vi "LVClasse_SurfaceFloat dtor.vi"(0 "SurfaceFloat in":refnum<class "SurfaceFloat.lvclass">, 11 "error in (no error)":errorcluster) -> (4 "SurfaceFloat out":refnum<class "SurfaceFloat.lvclass">, 15 "error out":errorcluster)   [LabVIEW 2020, in "SurfaceFloat.lvclass"]
doc: "Surface destructor.\n\n--------------------------------------------------------------------------------\n\n<B>surfaceIn </B> : Surface object.\n<B>surfaceOut </B> : Surface object.\n<B>ErrorIn </B> : Error\n<B>ErrorOut </B> : Error\n\n--------------------------------------------------------------------------------"
uses:
  SurfaceFloat.lvclass
  SurfaceFloat.lvclass/SurfaceFloat.ctl
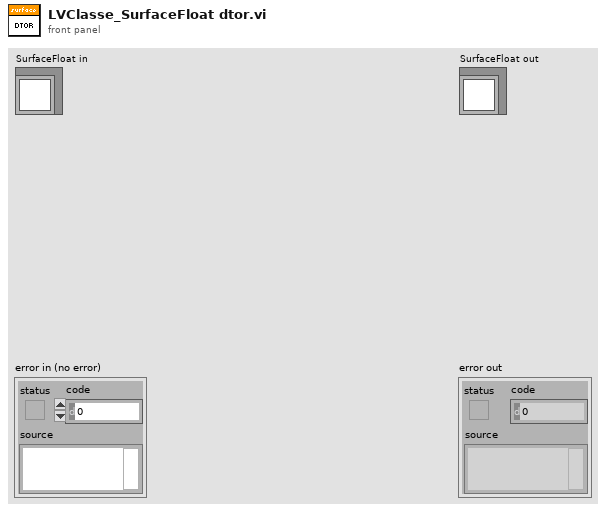
[diagram p1: front panel]
types:
  T1 = typedef "Handle creation.ctl" = enum16{"By ctor", "By write function"}
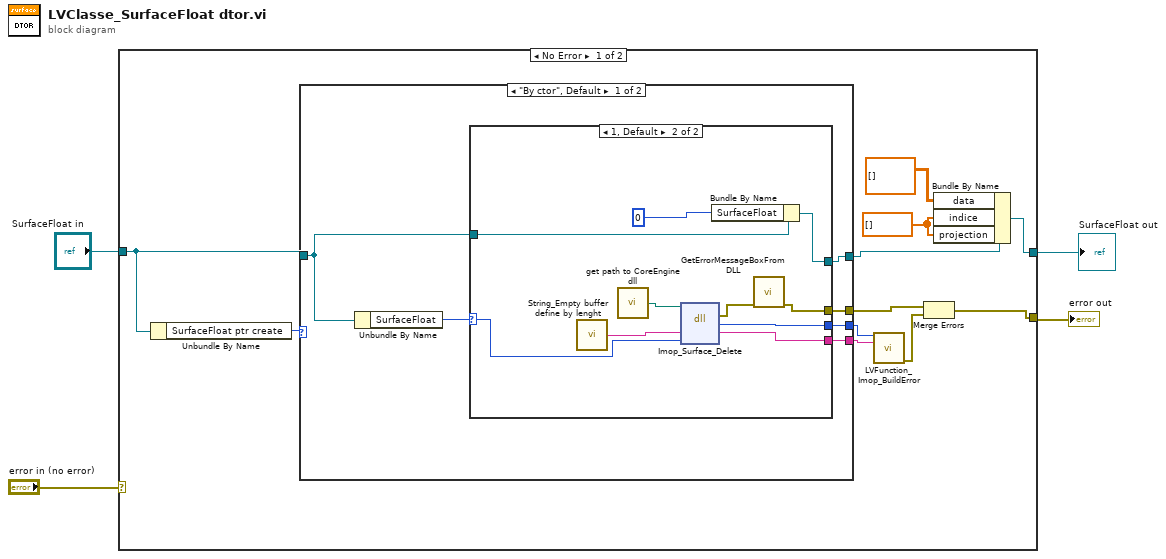
[diagram p0: block diagram]
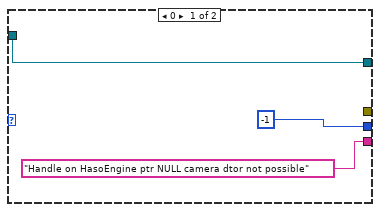
[diagram p2: hidden frame]
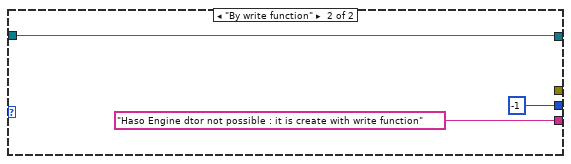
[diagram p3: hidden frame]
diagram:
  n1 = case shown="No Error" "error in (no error)" {
    selector: "error in (no error)" -> [_ w38]
    tunnel: "SurfaceFloat in" -> [w13 w39]
    tunnel: [w8 w39] -> w2
    tunnel: [w9 w38] -> w1
    frame No Error {
      w6 = sgl[] [] ("indice")
      n2 = Unbundle By Name(w13) -> ("SurfaceFloat ptr create"=w12:T1)
      n3 = case shown="\"By ctor\", Default" w12 {
        tunnel: [w21 "Haso Engine dtor not possible : it is create with write function" ("message")] -> w15
        tunnel: [w20 -1] -> w14
        tunnel: w13 -> [w18 w35]
        tunnel: [w19 w35] -> w7
        tunnel: [w16 _] -> w11
        frame "By ctor", Default {
          n4 = Unbundle By Name(w18) -> ("SurfaceFloat"=w17:i32)
          n5 = case shown="1, Default" w17 {
            selector: w17 -> [_ w31]
            tunnel: ["Handle on HasoEngine ptr NULL camera dtor not possible" ("message") w33] -> w21
            tunnel: [-1 w32] -> w20
            tunnel: w18 -> [w22 w27]
            tunnel: [w22 w26] -> w19
            tunnel: [_ w25] -> w16
            frame 0 {
            }
            frame 1, Default {
              n6 = call "String_Empty buffer define by lenght.vi"() -> ("Empty buffer"=w34:string)  [unwired: 1 in]
              n7 = call "get path to CoreEngine dll.vi"() -> ("path to c_interface_vc100.dll"=w30:path)  [unwired: 12 in, 3 out]
              n8 = dll-call lib="D:/soft/HASO_v3/SVN_trunk/ImOpCoreEngine4_LV2011/DLLs/c_interface_vc100.dll" fn="Imop_Surface_Delete"(path in=w30, "message"=w34, "surface"=w31) -> (error out=w29:errorcluster, "return type"=w32:i32, "message"=w33:string)  [unwired: 3 in, 1 out]
              n9 = Bundle By Name(cluster=w27, "SurfaceFloat"=u32 0 ("HasoEgine")) -> (w26:refnum<class "SurfaceFloat.lvclass">)
              n10 = call "GetErrorMessageBoxFromDLL.vi"("error IN"=w29) -> ("error OUT"=w25:errorcluster)  [unwired: 10 in]
            }
          }
        }
        frame "By write function" {
        }
      }
      n11 = call "LVFunction_Imop_BuildError.vi"("code"=w14, "String to Prepend to source (\"\")"=w15) -> ("error out"=w10:errorcluster)  [unwired: 13 in]
      n12 = Merge Errors(w11, w10) -> (w9:errorcluster)
      n13 = Bundle By Name(cluster=w7, "data"=sgl[][] [], "indice"=w6, "projection"=w6) -> (w8:refnum<class "SurfaceFloat.lvclass">)
    }
    frame Error {
    }
  }
  "error out" <- w1
  "SurfaceFloat out" <- w2
